vi "VI Scripting with Structures - For Loop.vi"   [LabVIEW 2019]
doc: "This example contains sample code demonstrating common VI Scripting navigational tasks relating to For Loops."
panel:
  # "Overview: Illustrates several ForLoop properties and methods used for inspecting and modifying For Loops with VI Scripting.\nInstructions:\nOpen the block diagram of this VI to see several examples of properties and methods related to For Loops and VI Scripting.\n\nNote: Browse the diagram of this example to learn about VI Scripting concepts. This example is not meant to be run."
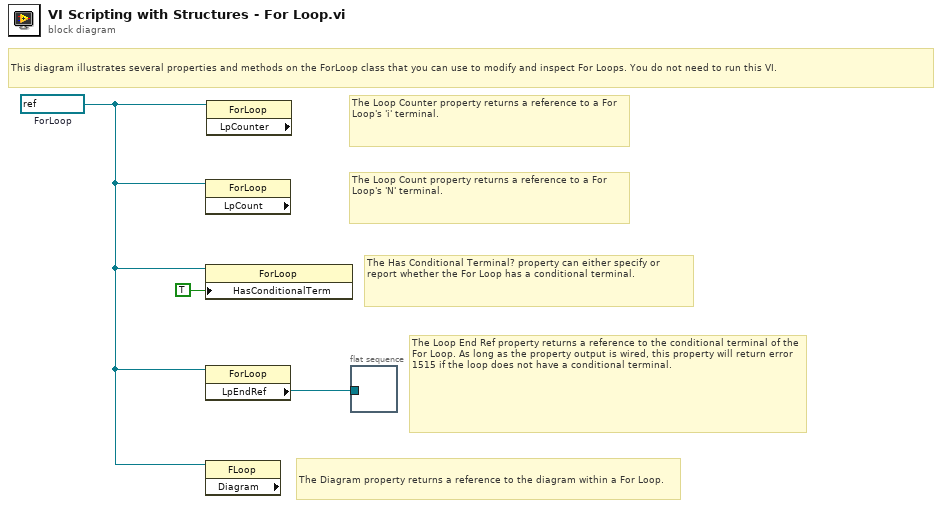
[diagram p0: block diagram]
diagram:
  w3 = refnum<vi> refnum  # ForLoop
  # "The Loop End Ref property returns a reference to the conditional terminal of the For Loop. As long as the property output is wired, this property will return error 1515 if the loop does not have a conditional terminal."
  # "The Diagram property returns a reference to the diagram within a For Loop."
  # "The Has Conditional Terminal? property can either specify or report whether the For Loop has a conditional terminal."
  # "The Loop Count property returns a reference to a For Loop's 'N' terminal."
  # "The Loop Counter property returns a reference to a For Loop's 'i' terminal."
  # "This diagram illustrates several properties and methods on the ForLoop class that you can use to modify and inspect For Loops. You do not need to run this VI."
  n1 = property class="ForLoop" props=["LpCount"](reference=w3) -> ()  [unwired: 1 in, 3 out]
  n2 = property class="ForLoop"(reference=w3, "HasConditionalTerm"=TRUE ("Has Conditional Terminal?")) -> ()  [unwired: 1 in, 2 out]
  n3 = property class="ForLoop"(reference=w3) -> ("LpEndRef"=w1:refnum<vi>)  [unwired: 1 in, 2 out]
  n4 = property class="FLoop" props=["Diagram"](reference=w3) -> ()  [unwired: 1 in, 3 out]
  n5 = property class="ForLoop" props=["LpCounter"](reference=w3) -> ()  [unwired: 1 in, 3 out]
  n6 = flat-sequence {
    tunnel: w1 -> [_]
    frame #0 {
    }
  }
